vi "StartTrial.vi"(8 "error in (no error)":errorcluster, 11 "TrialBasedExperiment in":refnum<class "DotMappingExperiment.lvclass">) -> (0 "error out":errorcluster, 3 "TrialBasedExperiment out":refnum<class "DotMappingExperiment.lvclass">)   [LabVIEW 2011, in "DotMappingExperiment.lvclass"]
uses:
  DotMappingExperiment.lvclass
  Trial Based Experiment Statechart/PassiveExperiment/PassiveExperiment.lvclass
  Matlab API/Matlab API.lvlib
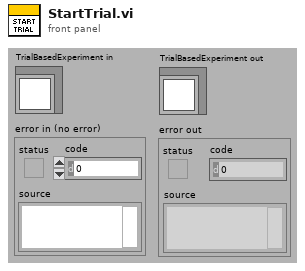
[diagram p1: front panel]
types:
  T1 = cluster{"Intertrial":dbl, "AcquireFixation":dbl, "HoldFixation":dbl, "DelayPeriod":dbl, "ResponsePeriod":dbl}
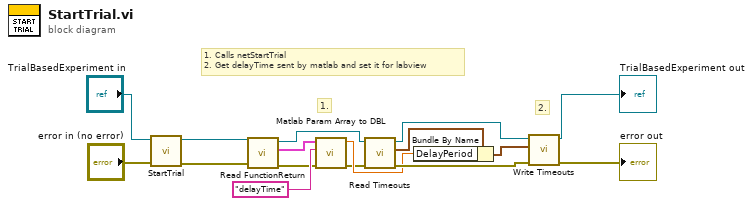
[diagram p0: block diagram]
diagram:
  # "1. Calls netStartTrial\n2. Get delayTime sent by matlab and set it for labview"
  # "2."
  # "1."
  n1 = call-parent "StartTrial.vi"("error in (no error)"="error in (no error)", "TrialBasedExperiment in"="TrialBasedExperiment in") -> ("error out"=w4:errorcluster, "TrialBasedExperiment out"=w5:refnum<class "DotMappingExperiment.lvclass">)  [unwired: 8 in]
  n2 = call-dynamic "Read FunctionReturn.vi"("error in (no error)"=w4, "MatlabExperiment in"=w5) -> ("error out"=w7:errorcluster, "FunctionReturn"=w1:cluster{"Name":string, "Data":variant}[], "MatlabExperiment out"=w14:refnum<class "DotMappingExperiment.lvclass">)  [unwired: 7 in]
  n3 = call "Matlab Param Array to DBL.vi"("error in (no error)"=w7, "Name"="delayTime", "Matlab Param Array"=w1) -> ("error out"=w6:errorcluster, "data"=w9:dbl)  [unwired: 7 in]
  n4 = call-dynamic "Read Timeouts.vi"("error in (no error)"=w6, "TrialBasedExperiment in"=w14) -> ("error out"=w12:errorcluster, "Timeouts"=w10:T1, "TrialBasedExperiment out"=w13:refnum<class "DotMappingExperiment.lvclass">)  [unwired: 7 in]
  n5 = Bundle By Name(cluster=w10, "DelayPeriod"=w9) -> (w8:T1)
  n6 = call-dynamic "Write Timeouts.vi"("error in (no error)"=w12, "Timeouts"=w8, "TrialBasedExperiment in"=w13) -> ("error out"=→"error out":errorcluster, "TrialBasedExperiment out"=→"TrialBasedExperiment out":refnum<class "DotMappingExperiment.lvclass">)  [unwired: 7 in]
